vi "per socket initialization.vi"(7 "id":i32, 8 "error in":errorcluster, 10 "upgrade data":T1, 11 "Websocket console plugin in":refnum<class "Websocket console plugin.lvclass">) -> (0 "error out":errorcluster, 3 "Websocket console plugin out":refnum<class "Websocket console plugin.lvclass">)   [LabVIEW 2013, in "Websocket console plugin.lvclass"]
uses:
  Websocket console plugin.lvclass
  HTTP responder/http upgrade data.ctl
  HTTP server/http request.ctl
  HTTP server/http method.ctl
  URI/url structure.ctl
  HTTP headers/http header data.ctl
  Websocket console plugin.lvclass/Websocket console plugin.ctl
  HTTP server/Basic HTTP server.lvclass
  HTTP responder/http responder.lvclass
  HTTP headers/http headers.lvlib
  URI/uniform resource locator.lvlib
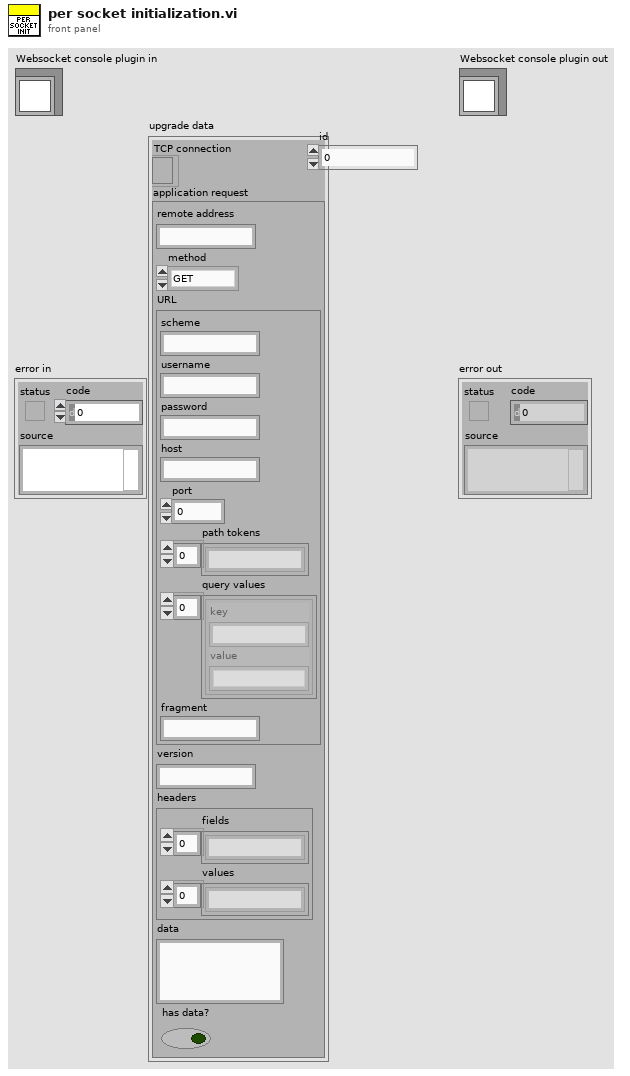
[diagram p1: front panel]
types:
  T1 = typedef "http responder.lvclass/http upgrade data.ctl" = cluster{"TCP connection":refnum<k5>, "application request":T2}
  T2 = typedef "Basic HTTP server.lvclass/http request.ctl" = cluster{"remote address":string, "method":T3, "URL":T4, "version":string, "headers":T5, "data":string, "has data?":bool}
  T3 = typedef "Basic HTTP server.lvclass/http method.ctl" = enum16{"GET", "POST", "PUT", "DELETE", "HEAD", "OPTIONS", "upgrade"}
  T4 = typedef "uniform resource locator.lvlib/url structure.ctl" = cluster{"scheme":string, "username":string, "password":string, "host":string, "port":u16, "path tokens":string[], "query values":cluster{"key":string, "value":string}[], "fragment":string}
  T5 = typedef "http headers.lvlib/http header data.ctl" = cluster{"fields":string[], "values":string[]}
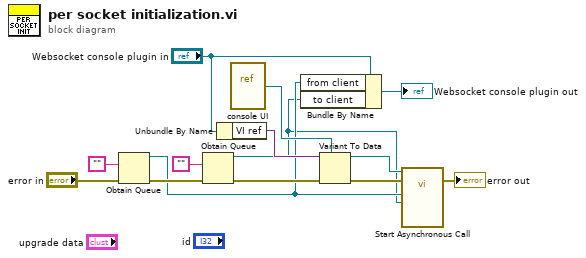
[diagram p0: block diagram]
diagram:
  n1 = Obtain Queue(element data type="", error in (no error)="error in") -> (queue out=w2:refnum<queue>, error out=w6:errorcluster)  [unwired: 3 in, 1 out]
  n2 = Obtain Queue(element data type="", error in (no error)=w6) -> (queue out=w1:refnum<queue>, error out=w5:errorcluster)  [unwired: 3 in, 1 out]
  n3 = Unbundle By Name("Websocket console plugin in") -> ("VI ref"=w14:variant)
  n4 = vi-ref "console UI.vi"() -> (w13:refnum<vi>)
  n5 = Bundle By Name(cluster="Websocket console plugin in", "from client"=w2, "to client"=w1) -> (→"Websocket console plugin out":refnum<class "Websocket console plugin.lvclass">)
  n6 = Variant To Data(error in=w5, type=w13, Variant=w14) -> (data=w10:refnum<vi>, error out=w11:errorcluster)
  n7 = call-by-ref "Start Asynchronous Call"(reference=w10, error in=w11, "to client"=w1, "from client"=w2) -> (error out=→"error out":errorcluster)  [unwired: 10 in, 1 out]
